vi "ATF Storage-Data Transfer Loop DD.vi"(9 "Data FIFO Ref":T1) -> ()   [LabVIEW 2022 SP3]
uses:
  RT Controls/ATF Storage-Data FIFO.ctl
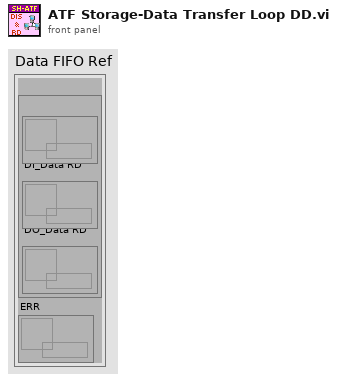
[diagram p1: front panel]
types:
  T1 = typedef "ATF Storage-Data FIFO.ctl" = cluster{"RD":cluster{"AI_V_Data RD":refnum<queue>, "DI_Data RD":refnum<queue>, "DO_Data RD":refnum<queue>}, "ERR":refnum<queue>}
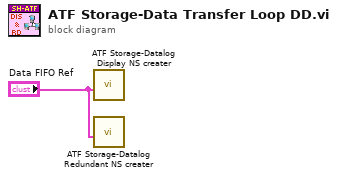
[diagram p0: block diagram]
diagram:
  n1 = call "ATF Storage-Datalog Display NS creater.vi"("Data FIFO Ref"="Data FIFO Ref") -> ()  [unwired: 11 in]
  n2 = call "ATF Storage-Datalog Redundant NS creater.vi"("Data FIFO Ref"="Data FIFO Ref") -> ()  [unwired: 11 in]
